vi "ConsoleHandlerLoop.vi"(8 "error in (no error)":errorcluster, 11 "ConsoleOutput in":refnum<class "ConsoleOutput.lvclass">) -> (0 "error out":errorcluster, 3 "ConsoleOutput out":refnum<class "ConsoleOutput.lvclass">)   [LabVIEW 2020, in "ConsoleOutput.lvclass"]
uses:
  ConsoleOutput.lvclass
  ConsoleOutput.lvclass/ConsoleOutput.ctl
  Lib/HSE-Logger/LogRecord/LogRecord.lvclass/LogRecord.ctl
  <vilib>/Utility/error.llb/DialogType.ctl
  Lib/HSE-Logger/LogRecord/Get Error.vi
  Lib/HSE-Logger/LogRecord/Get Message.vi
  Lib/HSE-Logger/LogRecord/LogRecord.lvclass
panel:
  out "Console Output":string
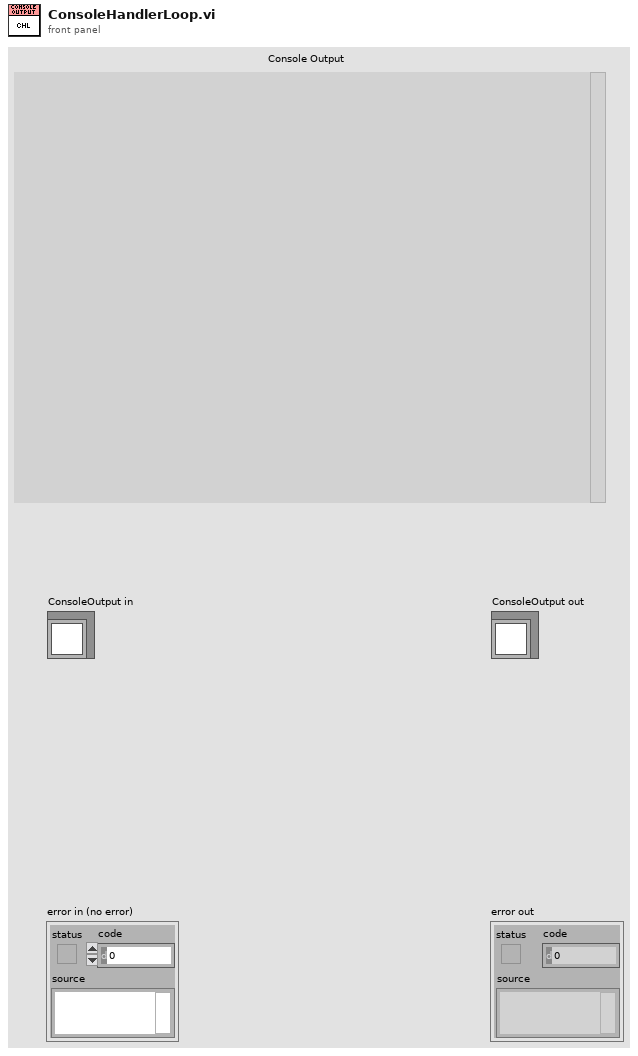
[diagram p1: front panel]
types:
  T1 = typedef "ConsoleOutput.lvclass/LogEventsRefum.ctl" = cluster{"LogRecord":refnum<user-event>, "Stop":refnum<user-event>}
  T2 = typedef "DialogType.ctl" = u16
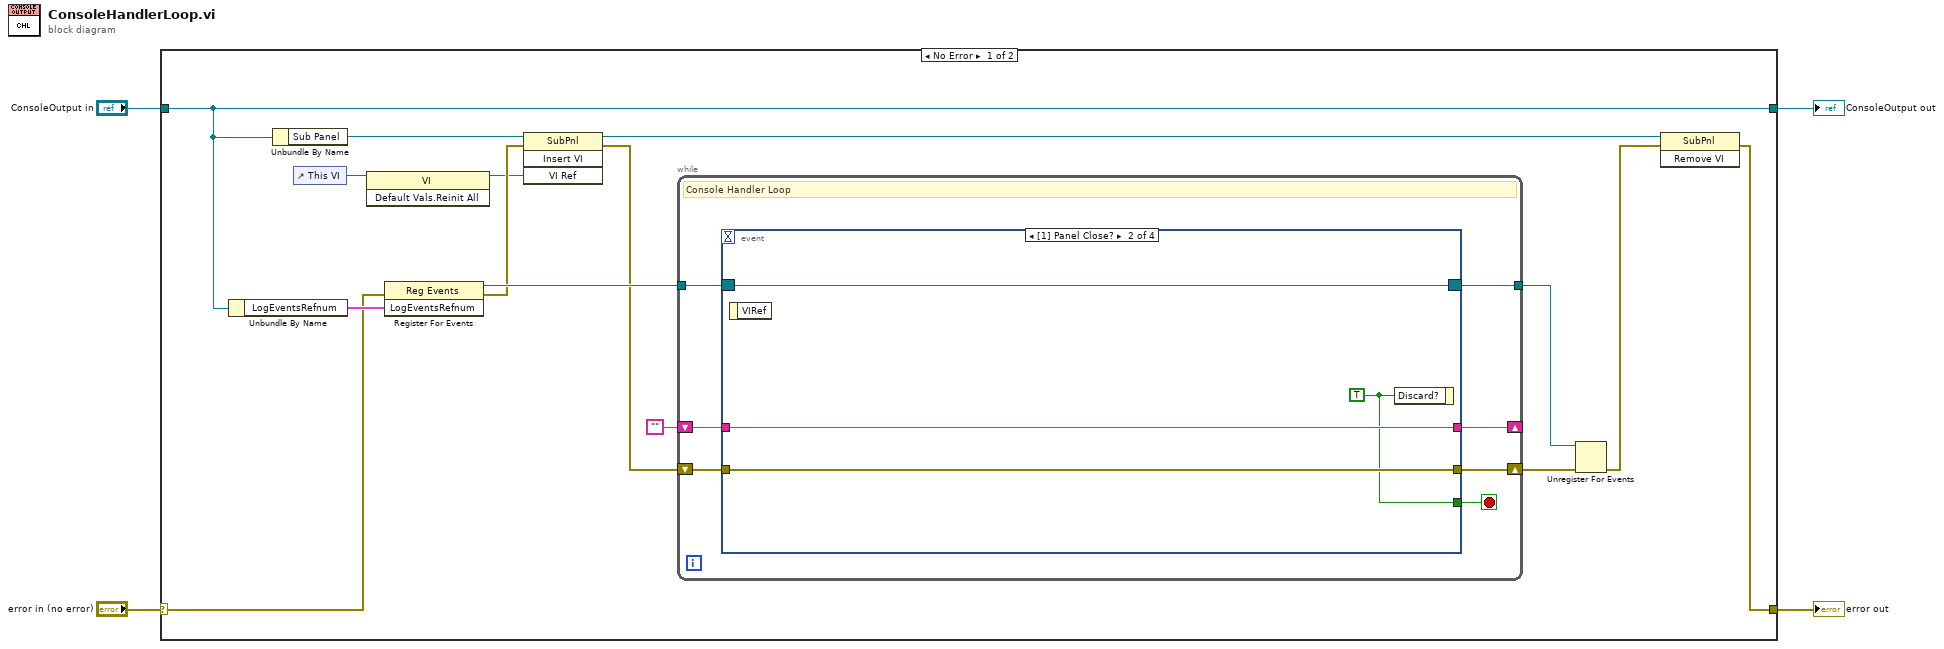
[diagram p0: block diagram]
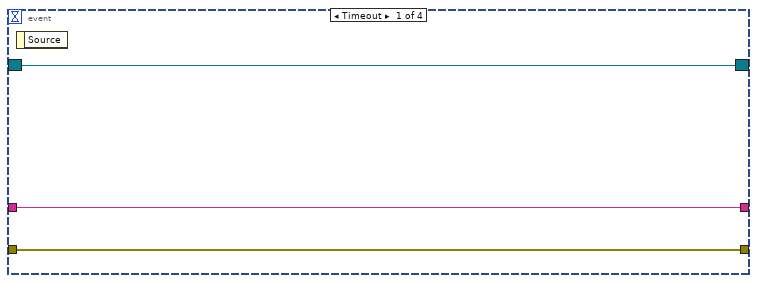
[diagram p2: hidden frame]
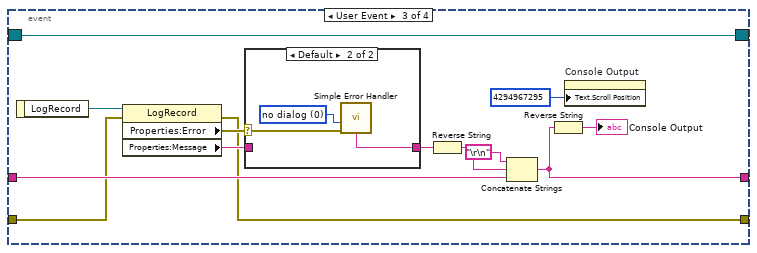
[diagram p3: hidden frame]
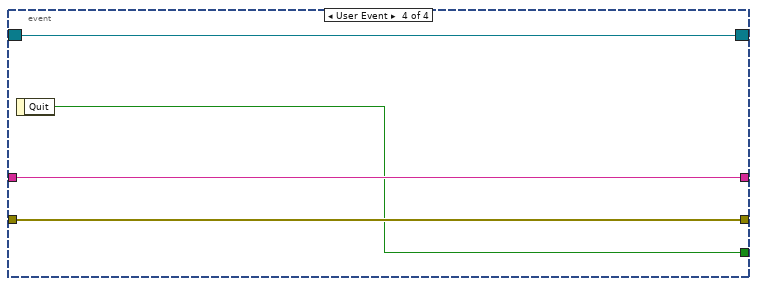
[diagram p5: hidden frame]
diagram:
  n1 = case shown="No Error" "error in (no error)" {
    selector: "error in (no error)" -> [w5 w56]
    tunnel: [w8 w56] -> w3
    tunnel: [w14 w55] -> w1
    tunnel: "ConsoleOutput in" -> [w14 w55]
    frame No Error {
      n2 = Unbundle By Name(w14) -> ("LogEventsRefnum"=w16:T1)
      n3 = Unbundle By Name(w14) -> ("Sub Panel"=w13:refnum<vi>)
      n4 = control-ref of="This VI"() -> (w7:refnum<vi>)
      n5 = invoke class="VI" method="Default Vals.Reinit All"(reference=w7) -> (reference out=w6:refnum<vi>)  [unwired: 2 in, 2 out]
      n6 = register-events(error in=w5, w16) -> (reference out=w18:refnum<event-registration>, error out=w12:errorcluster)  [unwired: 1 in]
      n7 = invoke class="SubPnl" method="Insert VI"(reference=w13, error in=w12, "VI Ref"=w6) -> (reference out=w11:refnum<vi>, error out=w9:errorcluster)  [unwired: 1 in, 2 out]
      n8 = while {
        shift-right: [w25] -> w17
        shift-left: w9 -> [w22]
        shift-right: [w23] -> _
        shift-left: "" -> [w26]
        tunnel: w18 -> [w24]
        tunnel: [w21] -> w15
        stop <- w20 stop-if-true
        # "Console Handler Loop"
        n9 = event shown="[1] Panel Close?" {
          selector: w24 -> [w28 w33 w40 w54]
          dyn-events: [w28 w33 w40 w54] -> w21
          timeout: _ -> [_ _ _ _]
          tunnel: w26 -> [w29 w32 w45 w53]
          tunnel: [w27 w31 w35 w52] -> w25
          tunnel: [w29 w32 w46 w53] -> w23
          tunnel: w22 -> [w27 w31 w36 w52]
          tunnel: [_ w30 _ w51] -> w20
          event Timeout {
            n10 = event-data() -> ()  [unwired: 1 in, 1 out]
          }
          event Panel Close? {
            w30 = TRUE
            n11 = event-data() -> ()  [unwired: 1 in, 1 out]
            n12 = event-data("Discard?"=w30) -> ()  [unwired: 1 in, 1 out]
          }
          event User Event {
            n13 = event-data() -> ("LogRecord"=w44:refnum<class "LogRecord.lvclass">)  [unwired: 1 in]
            n14 = property class="LogRecord"(reference=w44, error in=w36) -> (error out=w35:errorcluster, "Properties:Error"=w41:errorcluster, "Properties:Message"=w42:string)  [unwired: 1 out]
            n15 = case shown="Default" w41 {
              selector: w41 -> [_ w49]
              tunnel: [w47 w48] -> w43
              tunnel: w42 -> [w47 _]
              frame No Error {
              }
              frame Default {
                w50 = T2 0 items=["no dialog", "OK message", "continue or stop message", "OK message + warnings", "continue/stop + warnings"] ("type of dialog (OK msg:1)")
                n16 = call <vilib>:"Simple Error Handler.vi"("type of dialog (OK msg:1)"=w50, "error in (no error)"=w49) -> ("message"=w48:string)  [unwired: 3 in, 4 out]
              }
            }
            n17 = Reverse String(1:w43) -> (0:w38:string)
            n18 = Concatenate Strings("\r\n", w38, w45) -> (w46:string)
            n19 = Reverse String(1:w46) -> (0:→"Console Output":string)
            n20 = property on="Console Output" class="Str"("Text.Scroll Position"=u32 4294967295) -> ()  [unwired: 2 in, 2 out]
          }
          event User Event {
            n21 = event-data() -> ("Quit"=w51:bool)  [unwired: 1 in]
          }
        }
      }
      n22 = Unregister For Events(event registration refnum=w15, error in=w17) -> (error out=w10:errorcluster)
      n23 = invoke class="SubPnl" method="Remove VI"(reference=w11, error in=w10) -> (error out=w8:errorcluster)  [unwired: 1 in, 2 out]
    }
    frame Error {
    }
  }
  "error out" <- w3
  "ConsoleOutput out" <- w1
